vi "_test_toml.vi"(8 "error in (no error)":errorcluster) -> (0 "error out":errorcluster, 2 "tests":bool[](array[boolean]), 3 "passed":bool)   [LabVIEW 2017]
uses:
  58c06032-3e23-4c53-85e7-224e0a2187e2.vi
  toml_value_boolean.vi
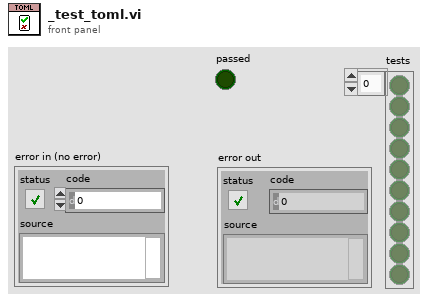
[diagram p1: front panel]
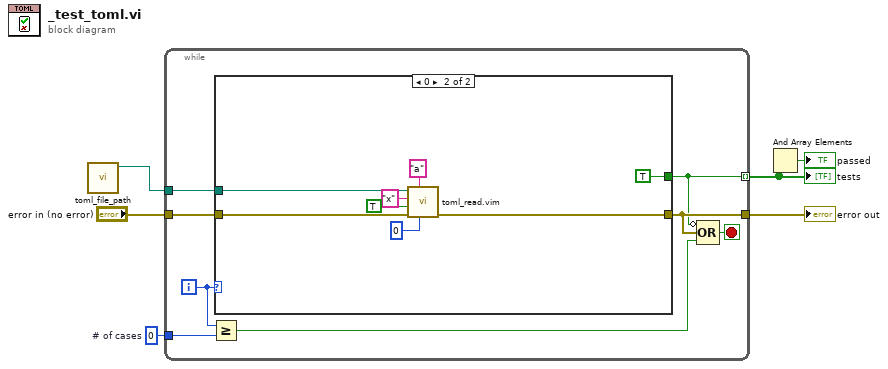
[diagram p0: block diagram]
diagram:
  w3 = 0  # # of cases
  n1 = call "toml_file_path.vi"() -> ("app toml path"=w6:path)  [unwired: 8 in, 3 out]
  n2 = while {
    tunnel: w6 -> [w14]
    tunnel: "error in (no error)" -> [w13]
    tunnel: [w12] -> w4
    tunnel: [w10] -> w2 mode=indexing
    tunnel: w3 -> [w8]
    i -> [w9]
    stop <- w11 stop-if-true
    n3 = Greater Or Equal?(x=w9, y=w8) -> (x >= y?=w7:bool)
    n4 = case shown="0" w9 {
      tunnel: w14 -> [_ w23]
      tunnel: w13 -> [w15 w22]
      tunnel: [w15 w21] -> w12
      tunnel: [_ TRUE] -> w10
      frame Default {
      }
      frame 0 {
        n5 = call "toml_read.vim"("modifiers"=u16 0 ("modifiers (default)"), "section [str,1d,pth]"="a", "error in (no error)"=w22, "default [any]"=TRUE, "key [str,1d,pth]"="x", "path in"=w23) -> ("error out"=w21:errorcluster)  [unwired: 2 in, 3 out]
      }
    }
    n6 = Compound Arithmetic op=OR(invert w10, w12, w7) -> (w11:bool)
  }
  "error out" <- w4
  "tests" <- w2
  n7 = And Array Elements(Boolean array=w2) -> (logical AND=→"passed":bool)
